vi "DAQ6363_ReadCounters.vi"(8 "ErrIn(No Err)":errorcluster caption="entrée d'erreur (pas d'erreur)", 10 "Count Period (ms)":u32=100, 11 "CntTask":refnum<k21> caption="Ch1CntTask") -> (0 "ErrOut":errorcluster caption="sortie d'erreur", 1 "Counts":u32, 2 "Counts/s":u32, 3 "CntTask Out":refnum<k21> caption="Ch1CntTaskOut", 4 "Period(ms)":u32, 5 "Jitter Warning":bool)   [LabVIEW 2019]
uses:
  <vilib>/DAQmx/read.llb/DAQmx Read (Counter U32 1Chan 1Samp).vi
  <vilib>/DAQmx/miscellaneous.llb/DAQmx Fill In Error Info.vi
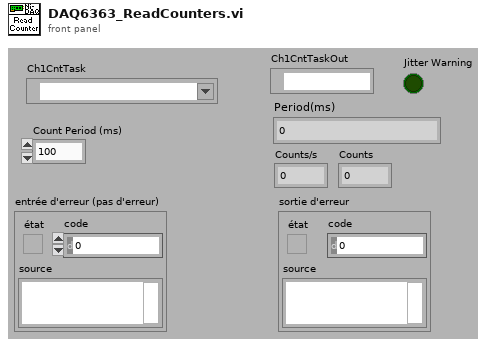
[diagram p1: front panel]
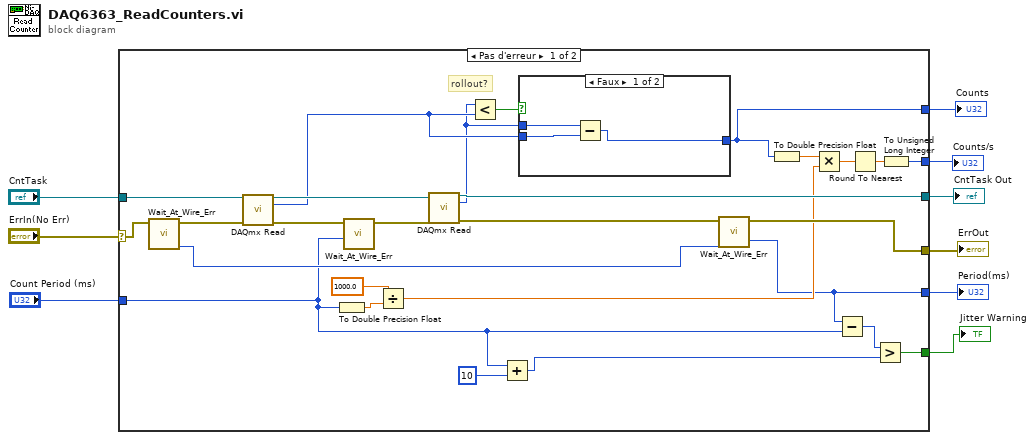
[diagram p0: block diagram]
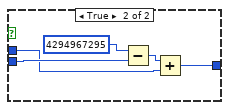
[diagram p2: hidden frame]
diagram:
  n1 = case shown="Pas d'erreur" "ErrIn(No Err)" {
    selector: "ErrIn(No Err)" -> [w35 w46]
    tunnel: [w28 w46] -> w8
    tunnel: "CntTask" -> [w36 w45]
    tunnel: [w34 w45] -> w6
    tunnel: [w20 _] -> w5
    tunnel: "Count Period (ms)" -> [w13 _]
    tunnel: [w15 _] -> w3
    tunnel: [w16 _] -> w2
    tunnel: [w10 _] -> w1
    frame No Error {
      # "rollout?"
      n2 = call <userlib>:"Wait_At_Wire_Err.vi"("error in (no error)"=w35) -> ("Clock(ms)"=w26:u32, "error out"=w31:errorcluster)  [unwired: 8 in, 1 out]
      n3 = call-poly <vilib>:"DAQmx Read.vi"("task/channels in"=w36, "error in"=w31) -> ("task out"=w30:refnum<k21>, "data"=w18:u32, "error out"=w33:errorcluster)  [unwired: 11 in]
      n4 = To Double Precision Float(number=w13) -> (double precision float=w24:dbl)
      n5 = call <userlib>:"Wait_At_Wire_Err.vi"("Wait (ms)"=w13, "error in (no error)"=w33) -> ("error out"=w32:errorcluster)  [unwired: 7 in, 2 out]
      n6 = Divide(x=1000.0 ("y"), y=w24) -> (x/y=w23:dbl)
      n7 = call-poly <vilib>:"DAQmx Read.vi"("task/channels in"=w30, "error in"=w32) -> ("task out"=w34:refnum<k21>, "data"=w17:u32, "error out"=w29:errorcluster)  [unwired: 11 in]
      n8 = Less?(x=w17, y=w18) -> (x < y?=w19:bool)
      n9 = Add(x=w13, y=u32 10) -> (x+y=w11:u32)
      n10 = case shown="Faux" w19 {
        tunnel: w18 -> [w38 w43]
        tunnel: w17 -> [w39 w41]
        tunnel: [w37 w40] -> w16
        frame False {
          n11 = Subtract(x=w39, y=w38) -> (x-y=w37:u32)
        }
        frame True {
          n12 = Subtract(x=u32 4294967295, y=w43) -> (x-y=w42:u32)
          n13 = Add(x=w42, y=w41) -> (x+y=w40:u32)
        }
      }
      n14 = call <userlib>:"Wait_At_Wire_Err.vi"("InitClock(ms)"=w26, "error in (no error)"=w29) -> ("error out"=w28:errorcluster, "Delta(ms)"=w15:u32)  [unwired: 7 in, 1 out]
      n15 = To Double Precision Float(number=w16) -> (double precision float=w22:dbl)
      n16 = Multiply(x=w22, y=w23) -> (x*y=w27:dbl)
      n17 = Subtract(x=w15, y=w13) -> (x-y=w14:u32)
      n18 = Round To Nearest(number=w27) -> (nearest integer value=w21:dbl)
      n19 = Greater?(x=w14, y=w11) -> (0:w10:bool)
      n20 = To Unsigned Long Integer(number=w21) -> (unsigned 32bit integer=w20:u32)
    }
    frame Error {
    }
  }
  "ErrOut" <- w8
  "CntTask Out" <- w6
  "Period(ms)" <- w3
  "Counts/s" <- w5
  "Counts" <- w2
  "Jitter Warning" <- w1
